vi "IR_ValueDisplay.vi"() -> ()   [LabVIEW 2019]
uses:
  WSCbot_V3_Toolkit.lvlibp/WSCBOTV3_Toolkit/Sensor/LowLevel/IR_Chanel.ctl
  WSCbot_V3_Toolkit.lvlibp
panel:
  out "Valtage":dbl[](array[numeric])=[1.5177045177045176, 1.5396825396825398, 0.020757020757020756, 0.020757020757020756, 0.31746031746031744, 0.28083028083028083, 1.514041514041514, 1.5433455433455434]
  out "Waveform Chart 8":dbl(graph)=1.514041514041514
  out "Waveform Chart 7":dbl(graph)=1.5433455433455434
  out "Waveform Chart 6":dbl(graph)=0.28083028083028083
  out "Waveform Chart 5":dbl(graph)=0.31746031746031744
  out "Waveform Chart 4":dbl(graph)=0.020757020757020756
  out "Waveform Chart 3":dbl(graph)=0.020757020757020756
  out "Waveform Chart 2":dbl(graph)=1.5396825396825398
  out "Waveform Chart":dbl(graph)=1.5177045177045176
  in  "Stop Button":bool
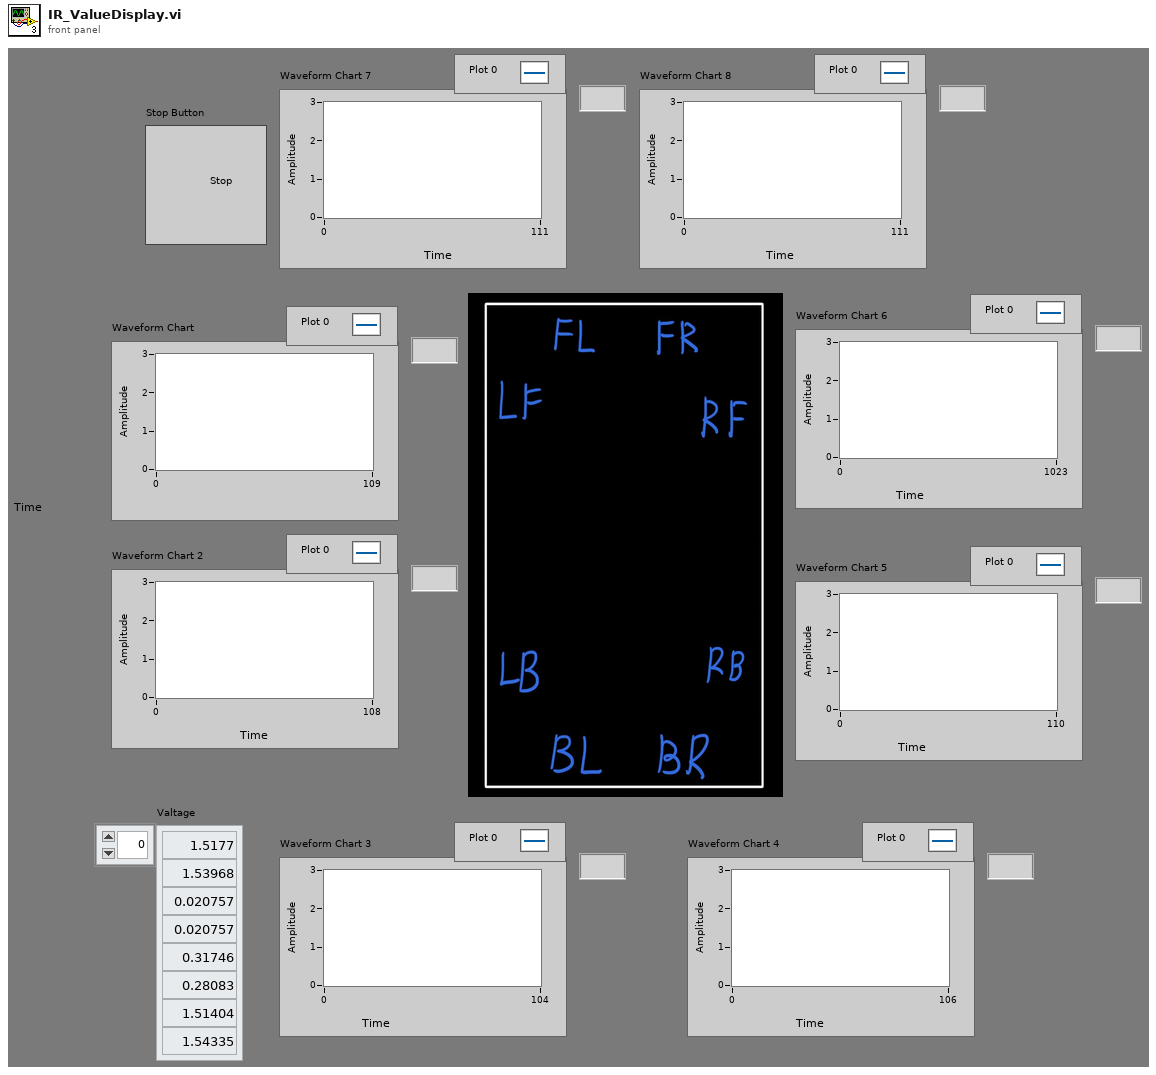
[diagram p1: front panel]
types:
  T1 = typedef "WSCbot_V3_Toolkit.lvlibp/IR_Chanel.ctl" = enum16{"IR_LF", "IR_LB", "IR_BL", "IR_BR", "IR_RB", "IR_RF", "IR_FR", "IR_FL"}
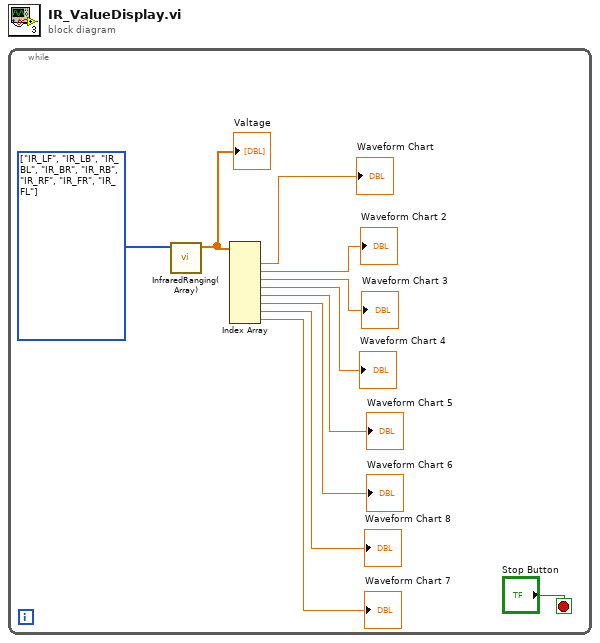
[diagram p0: block diagram]
diagram:
  n1 = while {
    stop <- "Stop Button" stop-if-true
    w10 = T1[] [enum."IR_LF", enum."IR_LB", enum."IR_BL", enum."IR_BR", enum."IR_RB", enum."IR_RF", enum."IR_FR", enum."IR_FL"] items=["IR_LF", "IR_LB", "IR_BL", "IR_BR", "IR_RB", "IR_RF", "IR_FR", "IR_FL"] ("IR_Chanel")
    n2 = call "InfraredRanging(Array).vi"("IR_Chanel"=w10) -> ("Valtage"=w9:dbl[])  [unwired: 9 in, 1 out]
    "Valtage" <- w9
    n3 = Index Array(array=w9) -> (element #1=→"Waveform Chart":dbl, element #2=→"Waveform Chart 2":dbl, element #3=→"Waveform Chart 3":dbl, element #4=→"Waveform Chart 4":dbl, element #5=→"Waveform Chart 5":dbl, element #6=→"Waveform Chart 6":dbl, element #7=→"Waveform Chart 8":dbl, element #8=→"Waveform Chart 7":dbl)  [unwired: 8 in]
  }
